vi "Write Setting.vi"(8 "error in (no error)":errorcluster, 9 "Tag Attribute":variant, 10 "Tag Name":string, 11 "Save Restore Settings in":refnum<class "Save Restore Settings.lvclass">) -> (0 "error out":errorcluster, 3 "Save Restore Settings out":refnum<class "Save Restore Settings.lvclass">)   [LabVIEW 2016, in "Save Restore Settings.lvclass"]
uses:
  <userlib>/_MGI/Application Control/MGI Save Restore Settings/Save Restore Settings.lvclass
  <userlib>/_MGI/Application Control/MGI Save Restore Settings/Save Restore Settings.lvclass/Save Restore Settings.ctl
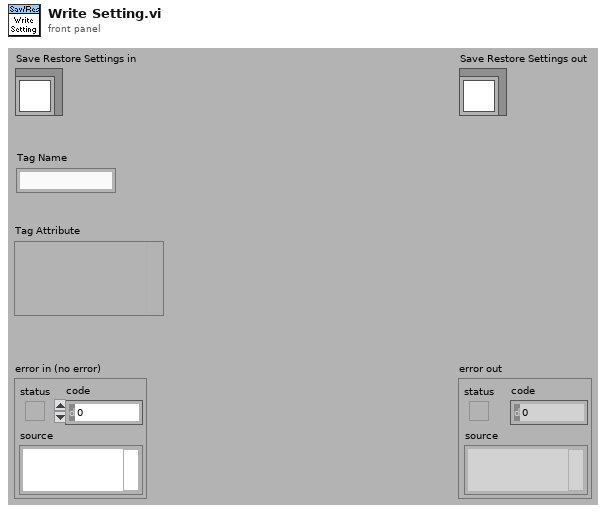
[diagram p1: front panel]
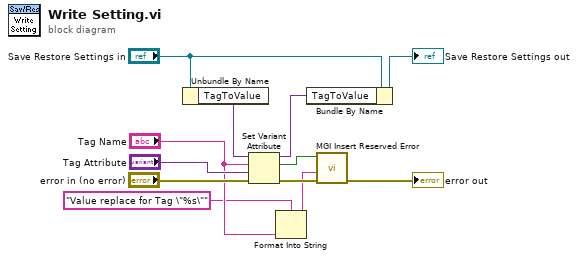
[diagram p0: block diagram]
diagram:
  n1 = Unbundle By Name("Save Restore Settings in") -> ("TagToValue"=w9:variant)
  n2 = Set Variant Attribute(Variant=w9, name="Tag Name", value="Tag Attribute", error in="error in (no error)") -> (Variant out=w6:variant, replaced=w7:bool, error out=w8:errorcluster)
  n3 = Format Into String(format string="Value replace for Tag \"%s\"", "Tag Name") -> (resulting string=w2:string)  [unwired: 2 in, 1 out]
  n4 = Bundle By Name(cluster="Save Restore Settings in", "TagToValue"=w6) -> (→"Save Restore Settings out":refnum<class "Save Restore Settings.lvclass">)
  n5 = call <userlib>:"MGI Insert Reserved Error.vi"("Error In"=w8, "Error Description"=w2, "Error? (T)"=w7) -> ("Error Out"=→"error out":errorcluster)  [unwired: 8 in]
